vi "ATE_NS_DL_cal.vi"() -> ()   [LabVIEW 2009]
doc: "Use this template to build a producer/consumer design pattern with events to produce queue items. Use this design pattern instead of the User Interface Event Handler pattern for user interfaces when you want to execute code asynchronously in response to an event without slowing the user interface responsiveness."
uses:
  Rvp8PowerData.ctl
panel:
  in  "70 dB Attn":i32=70 min=0 max=70 step=10
  in  "READY":bool
  out "Instructions":string="Noise Source Dummy Load Calibration\n\n1 - Disable or turn off transmitter\n2 - Stow Antenna (point vertically)\n3 - Turn off all florescnt lights\n3 - Start the labview program by clicking the Run arrow\n     (left most button under  drop down menues)\n     start cycle time about 35 seconds\n4 - Wait for the red 'BUSY' light to change to green 'READY'\n     All the control buttons on the control panel are active.\n5 - Select the noise source, its state (ON/OFF) and the wave\n     guide termination.\n6 - Calibrate with the red  'Calibrate' button\n      calibration cycle time is less than 1 minute\n7 - Exit the program with the red 'EXIT' button\n      exit cycle time about 20 seconds\n\nHints:\nWait for the green 'READY' light before clicking buttons\nAll the status leds on the 'Status' tab should be green during a calibration.\nThe antenna noise source does not work with the wave guide\ntermination in the 'Dummy Load' position."
  in  "Configuration 1":bool
  out "Cal Output File":path
  out "Cal file name":string
  in  "Cal data directory":string="/home/operator/ate/data/rvp8_cal"
  in  "Set SigGen":bool
  in  "Initialize":bool
  in  "70 dB":bool
  in  "121 dB":bool
  in  "Switches":bool
  in  "Calibrate":bool
  in  "Stop":bool
  in  "ATE TABS":enum32{"Status", "Controls"}(tab)
  out "ATE Switch Status":T1
  out "RVP8 Power":T2 {"time" format="%<%H:%M:%S\n%Y/%m/%d>T"}
  out "121dB\nAttenuators":bool[](array[boolean])
  out "121 Verified":bool
  out "Inside Noise Box":bool
  in  "WG3 MS":bool
  in  "WG3 T":bool
  out "WG3":bool
  in  "WG2 MS":bool
  in  "WG2 T":bool
  out "WG2":bool
  in  "WG1 MS":bool
  in  "WG1 T":bool
  out "WG1":bool
  in  "WG5 ANT":bool
  in  "WG5 DL":bool
  out "WG5":bool
  in  "WG4 ANT":bool
  in  "WG4 DL":bool
  out "WG4":bool
  out "Outside Noise Box":bool
  out "XmStat":bool=TRUE
  in  "ATE Switches":T3={"Reversing Switch"=enum."Normal Function", "IO Switch #1 Input"=enum."NONE", "IO Switch #1 Output"=enum."NONE", "IO Switch #2 Input"=enum."NONE", "IO Switch #2 Output"=enum."NONE", "Signal Out Input"=enum."NONE", "Signal Out Output"=enum."NONE", "Signal Source Input"=enum."NONE", "Signal Source Output"=enum."NONE", "Power Meter Switch Input"=enum."NONE", "Pouer Meter Switch Output"=enum."NONE", "Amplifier Switch"=enum."Include Amp"}
  in  "DataSource":bool=TRUE
  in  "Measurements":i32=10
  in  "121 dB Atten":i32 min=0 max=121 step=1
  in  "NS_on/off":bool
  in  "Wave Guide Termination":bool
  in  "NoiseSource":u16(ring) items=["Inside Noise Source", "Outside Noise Source", "Agilent Noise Inside", "Agilent Noise Outside"]
  out "P-State":string
  out "C-State":string
  in  "BUSY":bool
  # "ATE Noise Source Calibration"
  # "1 dB"
  # "2 dB"
  # "4 dB"
  # "4 dB"
  # "10 dB"
  # "20 dB"
  # "40 dB"
  # "40 dB"
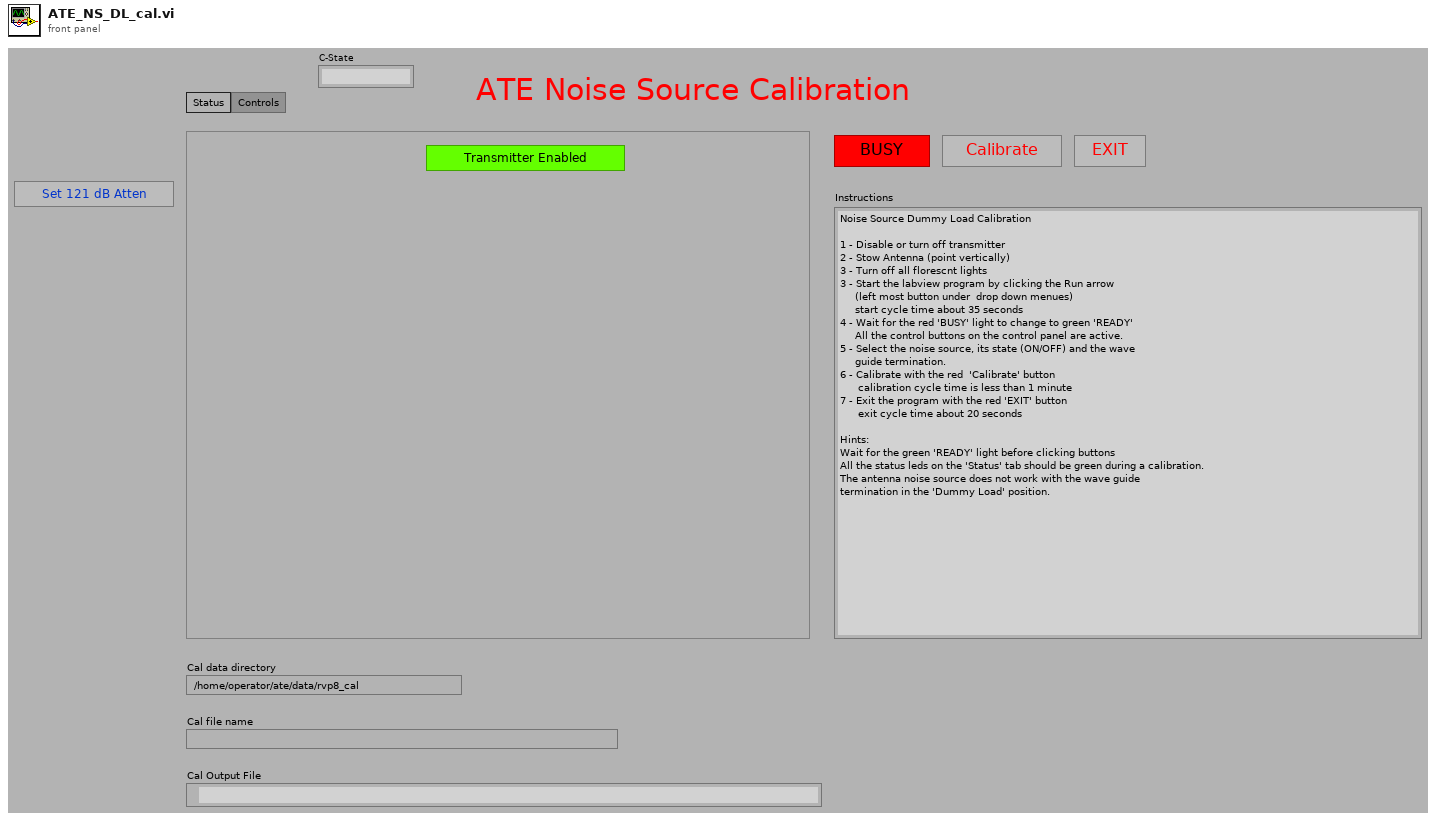
[diagram p1: front panel]
types:
  T1 = cluster{"Reversing Switch ":bool, "IO Switch #1":bool, "IO Switch #2":bool, "Signal Out":bool, "Signal Source":bool, "Power Meter":bool, "Amp By Pass":bool}
  T2 = typedef "Rvp8PowerData.ctl" = cluster{"success":bool, "time":dbl, "el":dbl, "az":dbl, "dbm0":dbl, "dbm1":dbl, "dbmHc":dbl, "dbmHx":dbl, "dbmVc":dbl, "dbmVx":dbl}
  T3 = cluster{"Reversing Switch":enum16{"Normal Function", "Reversing Function"}, "IO Switch #1 Input":enum16{"NONE", "AHR (J2)", "Splitter", "Signal Out Switch (S3)", "Reversing Switch"}, "IO Switch #1 Output":enum16{"NONE", "AHR (J2)", "Delay Device (S4)", "Power Meter Switch (S5)", "Reversing Switch"}, "IO Switch #2 Input":enum16{"NONE", "AVR (J3)", "Splitter", "Signal Out Switch (S3)", " 2W Term (TM1)", "Reversing Switch"}, "IO Switch #2 Output":enum16{"NONE", "AVR (J3)", "Signal Out Switch (S3)", "Power Meter Switch (S5)", "Reversing Switch", "2W Term (TM1)"}, "Signal Out Input":enum16{"NONE", "Amp Bypass Switch (S6)", "IO Switch #1 (S1)", "IO Switch #2 (S2)", "2W Term (TM3)"}, "Signal Out Output":enum16{"NONE", "2 Watt Term (TM3)", "Splitter", "Power Meter Switch (S5)"}, "Signal Source Input":enum16{"NONE", "Delay Device", "Signal Generator (J7)", "Inside Noise Box NF (J5)", "2W Term (TM3)"}, "Signal Source Output":enum16{"NONE", "Amp Bypass Switch", "Test Pulse Generator", "Power Meter Switch (S5)"}, "Power Meter Switch Input":enum16{"NONE", "IO Switch #1 (S1)", "Signal Source Switch (S4)", "Signal Out Switch (S3)", "IO Switch #2 (S2)", "TXH-TXV Switch (J8)"}, "Pouer Meter Switch Output":enum16{"NONE", "Power Meter (J6)"}, "Amplifier Switch":enum16{"Bypass Amp", "Include Amp"}}
  T4 = cluster{"Frequency (GHz)":dbl, "RF Power (dBm)":dbl, "RF ON/OFF":bool}
  T5 = enum16{"open", "replace", "create", "open or create", "replace or create", "replace or create with confirmation"}
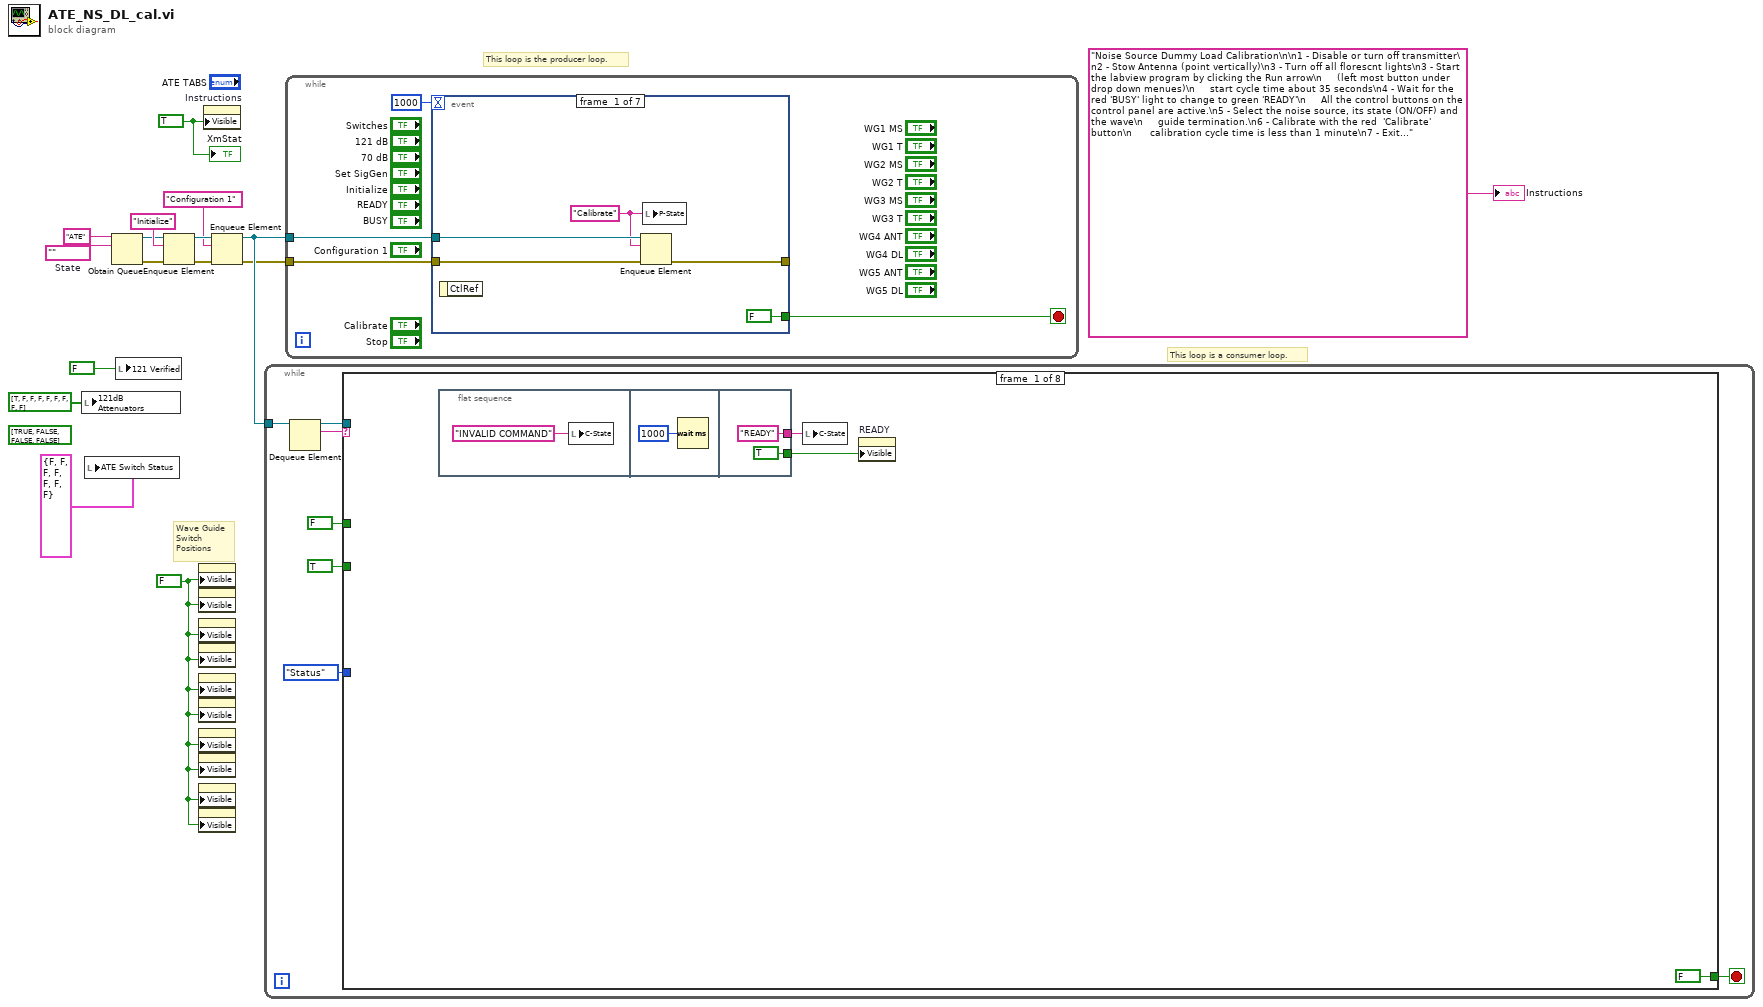
[diagram p0: block diagram]
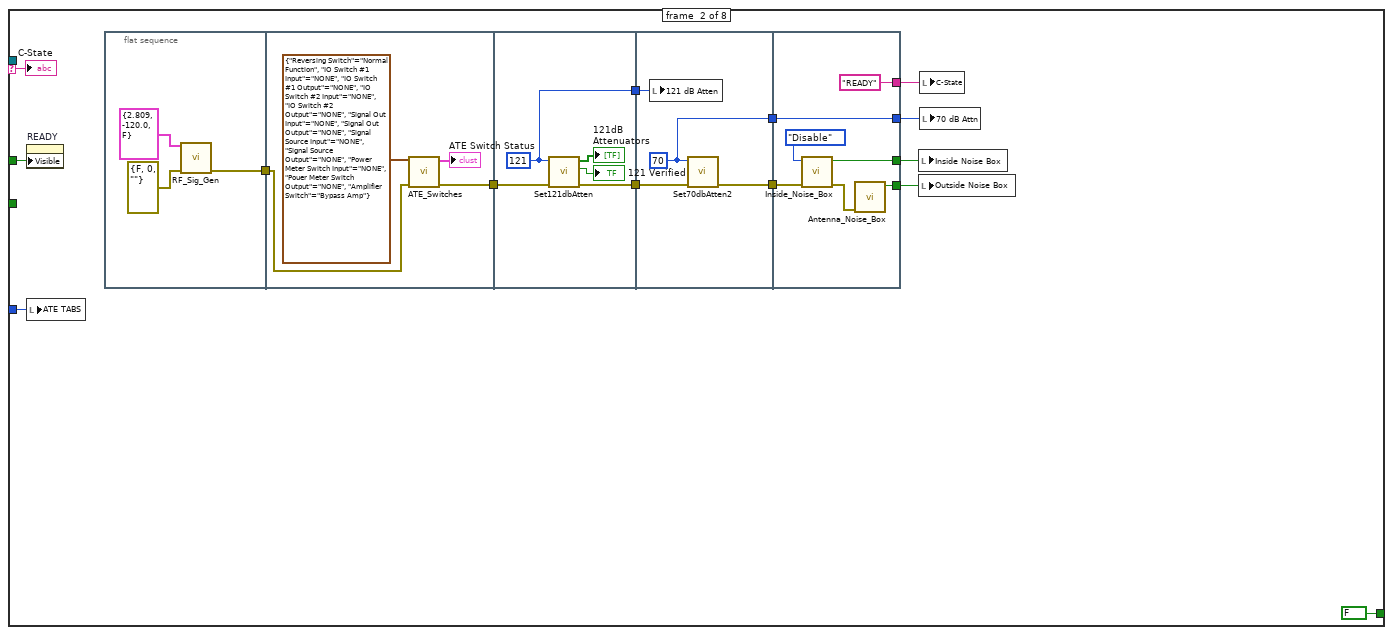
[diagram p2: hidden frame]
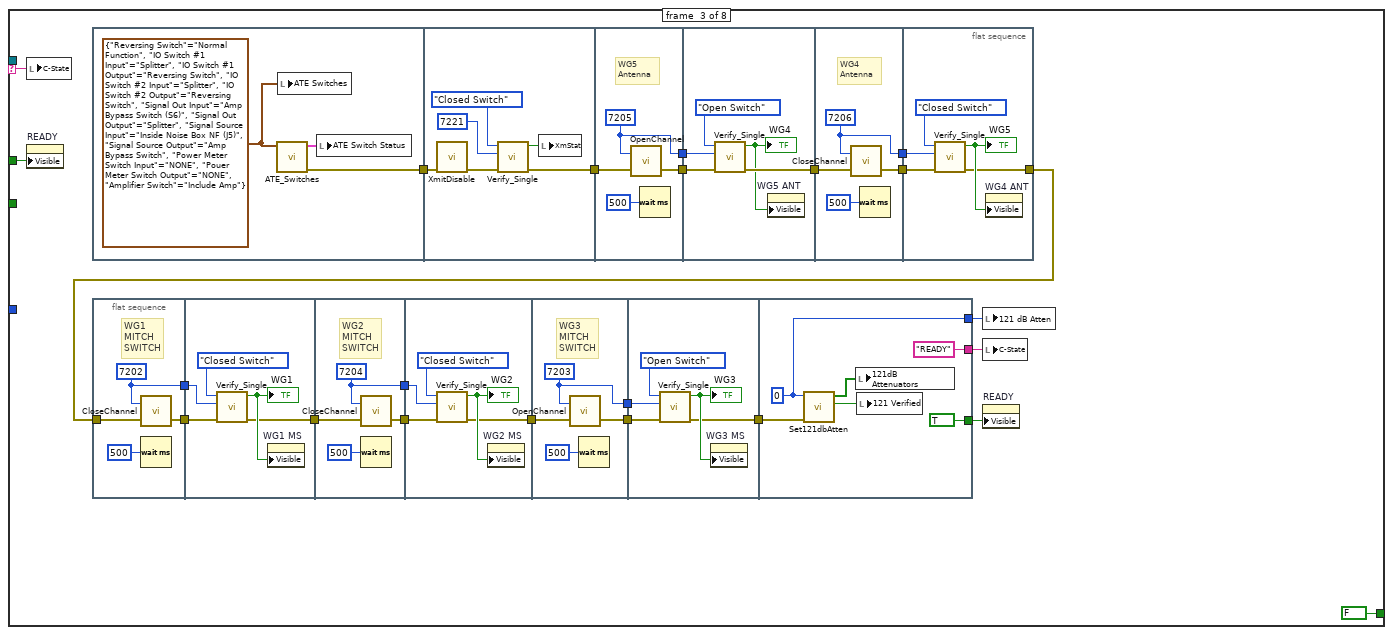
[diagram p3: hidden frame]
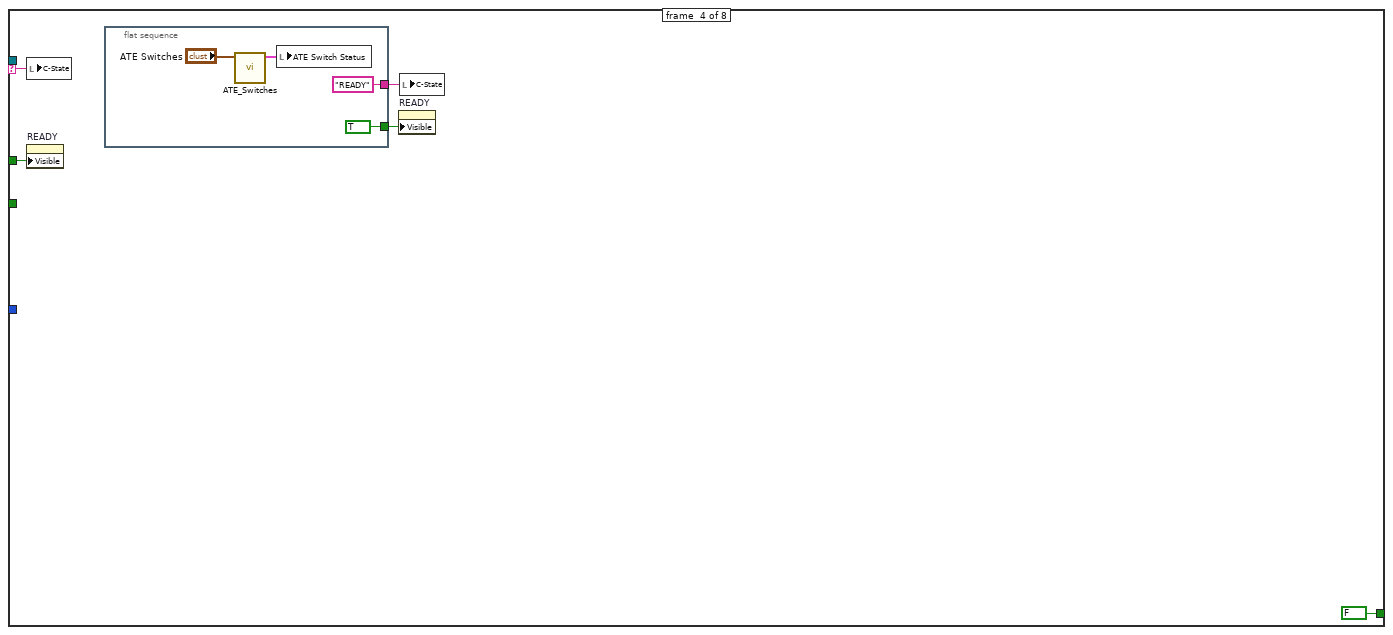
[diagram p4: hidden frame]
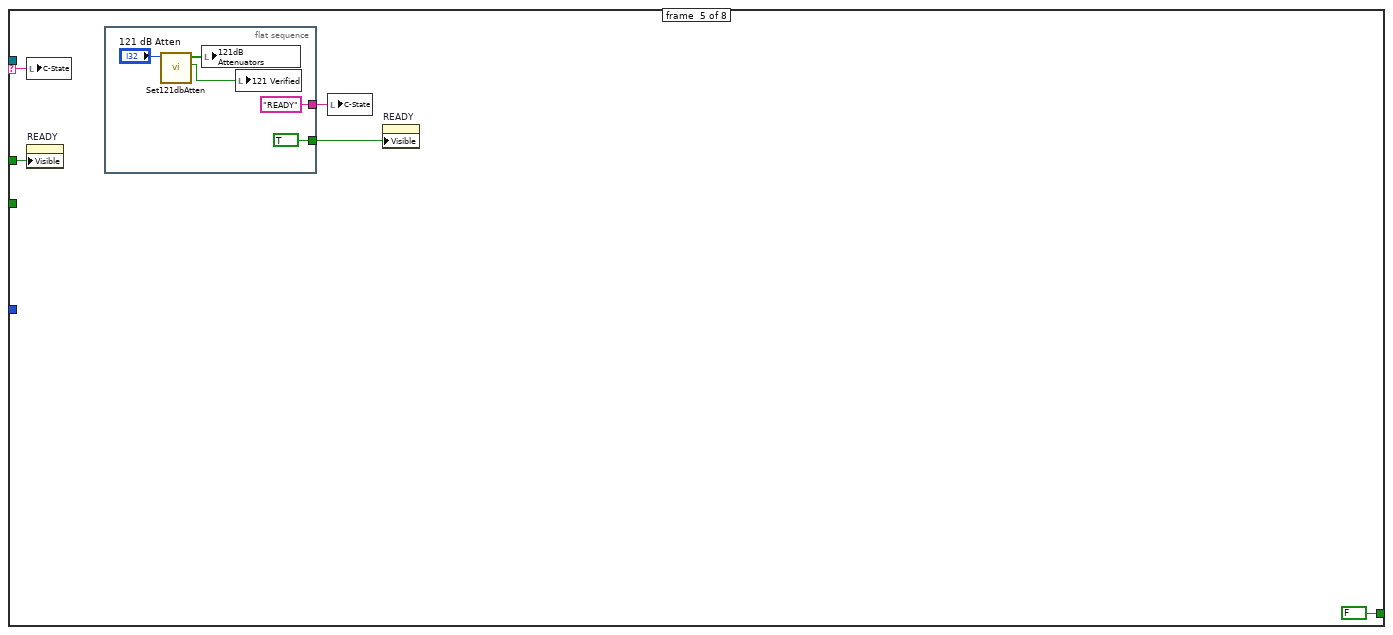
[diagram p5: hidden frame]
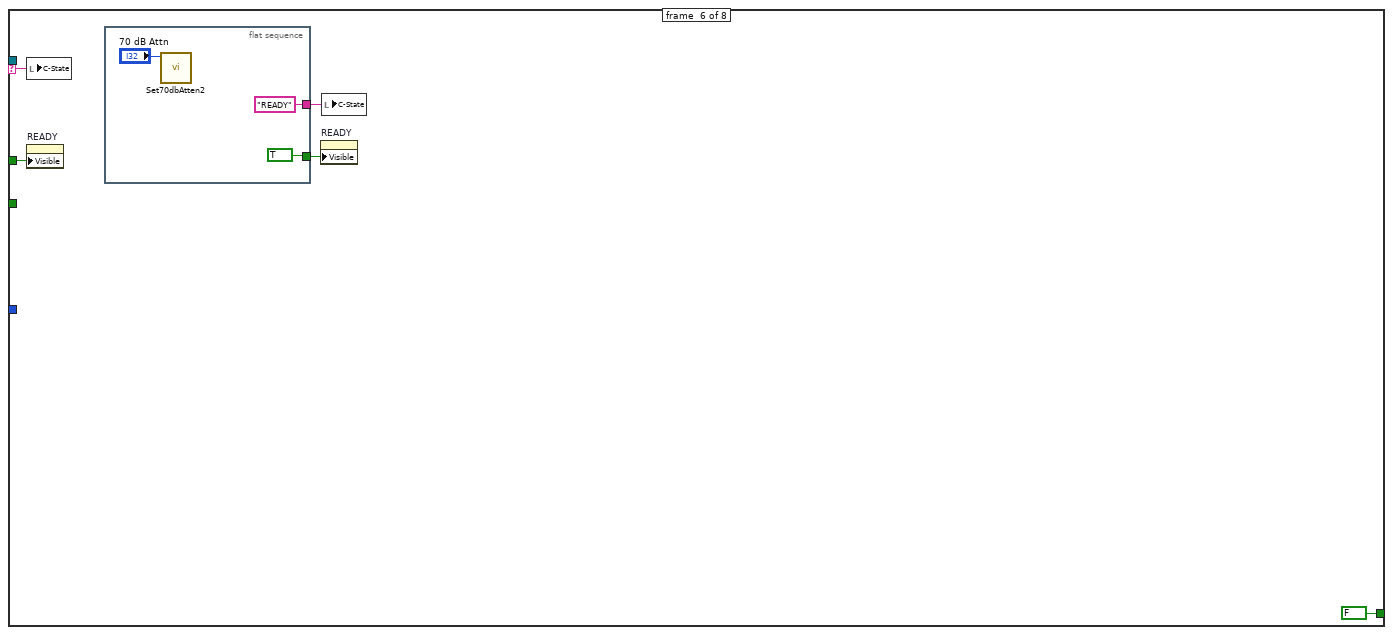
[diagram p6: hidden frame]
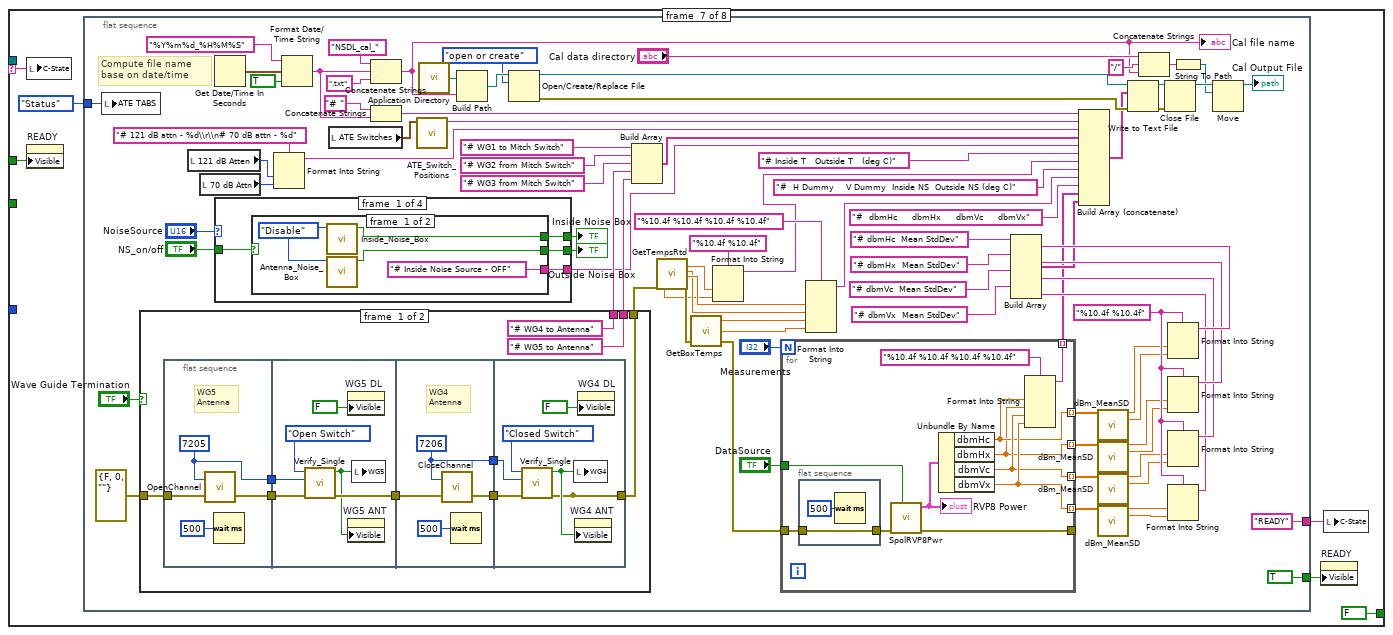
[diagram p7: hidden frame]
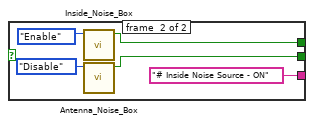
[diagram p8: hidden frame]
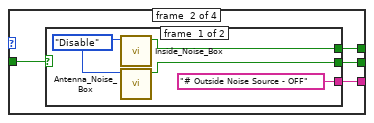
[diagram p9: hidden frame]
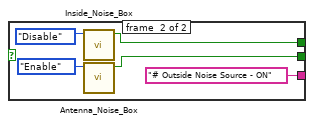
[diagram p10: hidden frame]
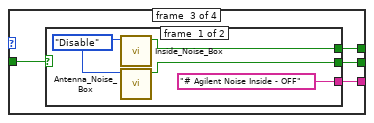
[diagram p11: hidden frame]
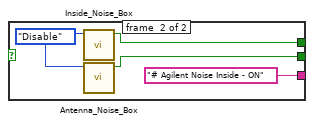
[diagram p12: hidden frame]
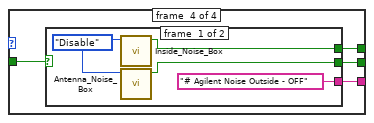
[diagram p13: hidden frame]
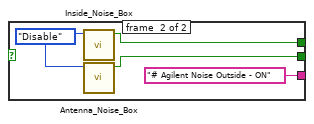
[diagram p14: hidden frame]
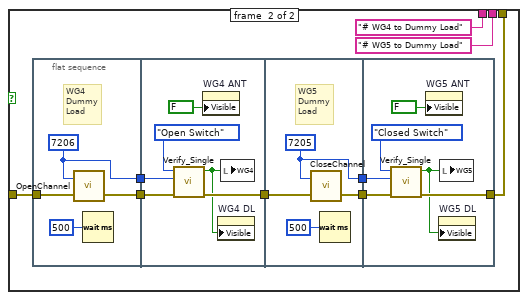
[diagram p15: hidden frame]
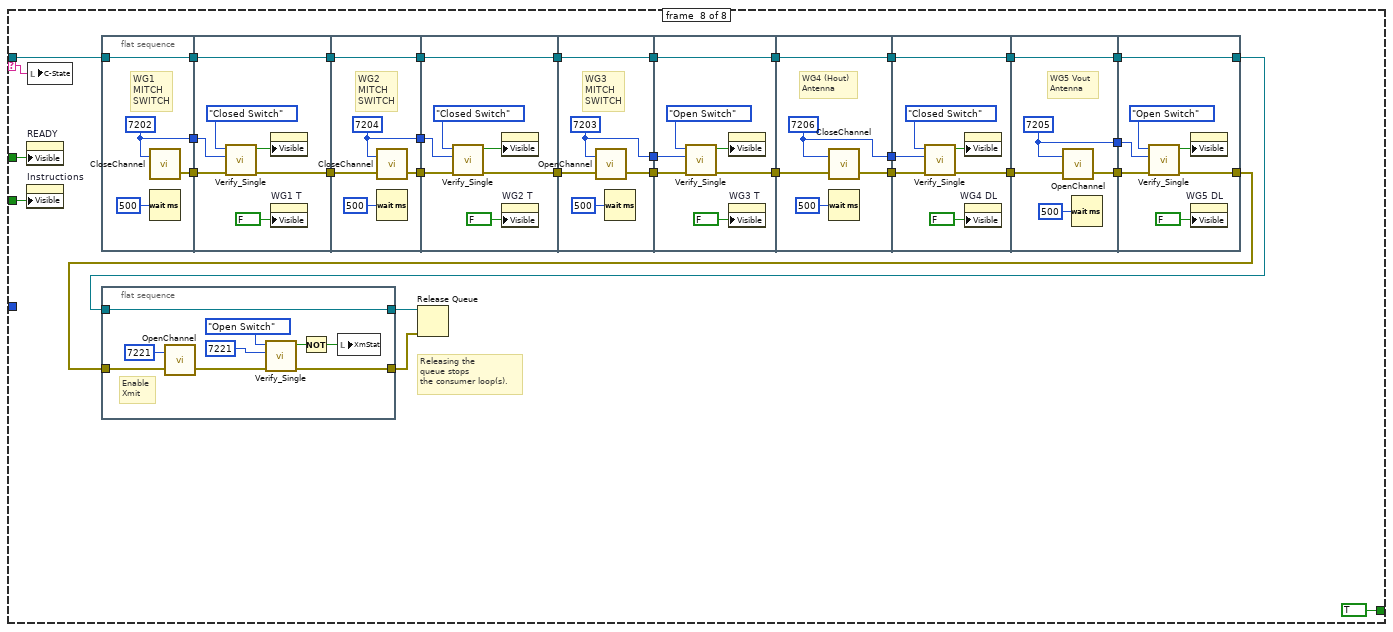
[diagram p16: hidden frame]
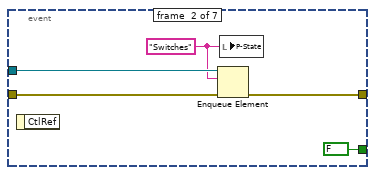
[diagram p17: hidden frame]
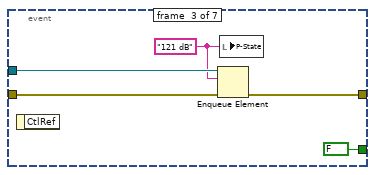
[diagram p18: hidden frame]
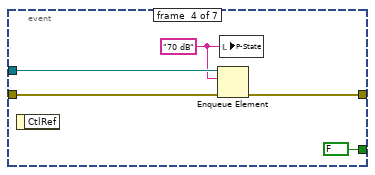
[diagram p19: hidden frame]
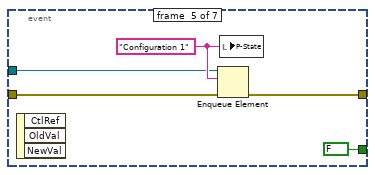
[diagram p20: hidden frame]
diagram:
  w6 = FALSE ("Visible")
  w1 = TRUE ("Visible")
  (unwired) bool[] [TRUE, FALSE, FALSE, FALSE] ("70dB\nAttenuators")
  w16 = ""  # State
  # "Wave Guide\nSwitch\nPositions"
  # "This loop is the producer loop."
  # "This loop is a consumer loop."
  n1 = local write "121dB\nAttenuators"(bool[] [TRUE, FALSE, FALSE, FALSE, FALSE, FALSE, FALSE, FALSE, FALSE] ("121dB\nAttenuators")) -> ()
  n2 = local write "ATE Switch Status"(T1 {"Reversing Switch "=FALSE, "IO Switch #1"=FALSE, "IO Switch #2"=FALSE, "Signal Out"=FALSE, "Signal Source"=FALSE, "Power Meter"=FALSE, "Amp By Pass"=FALSE} ("ATE Switch Status")) -> ()
  n3 = Obtain Queue(name (unnamed)="ATE", element data type=w16) -> (queue out=w13:refnum<queue>, error out=w12:errorcluster)  [unwired: 3 in, 1 out]
  n4 = local write "121 Verified"(FALSE ("70 Verfied")) -> ()
  n5 = Enqueue Element(queue=w13, element="Initialize", error in (no error)=w12) -> (queue out=w7:refnum<queue>, error out=w4:errorcluster)  [unwired: 1 in, 1 out]
  n6 = property on="WG1 MS" class="Bool"("Visible"=w6) -> ()  [unwired: 2 in, 2 out]
  n7 = property on="WG1 T" class="Bool"("Visible"=w6) -> ()  [unwired: 2 in, 2 out]
  n8 = property on="WG2 MS" class="Bool"("Visible"=w6) -> ()  [unwired: 2 in, 2 out]
  n9 = property on="WG2 T" class="Bool"("Visible"=w6) -> ()  [unwired: 2 in, 2 out]
  n10 = property on="WG3 MS" class="Bool"("Visible"=w6) -> ()  [unwired: 2 in, 2 out]
  n11 = property on="WG3 T" class="Bool"("Visible"=w6) -> ()  [unwired: 2 in, 2 out]
  n12 = property on="WG4 ANT" class="Bool"("Visible"=w6) -> ()  [unwired: 2 in, 2 out]
  n13 = property on="WG4 DL" class="Bool"("Visible"=w6) -> ()  [unwired: 2 in, 2 out]
  n14 = property on="WG5 ANT" class="Bool"("Visible"=w6) -> ()  [unwired: 2 in, 2 out]
  n15 = property on="WG5 DL" class="Bool"("Visible"=w6) -> ()  [unwired: 2 in, 2 out]
  n16 = property on="Instructions" class="Str"("Visible"=w1) -> ()  [unwired: 2 in, 2 out]
  n17 = Enqueue Element(queue=w7, element="Configuration 1", error in (no error)=w4) -> (queue out=w5:refnum<queue>, error out=w3:errorcluster)  [unwired: 1 in, 1 out]
  n18 = while {
    tunnel: w5 -> [w23]
    stop <- w20 stop-if-true
    n19 = Dequeue Element(queue=w23) -> (queue out=w21:refnum<queue>, element=w22:string)  [unwired: 2 in, 2 out]
    n20 = case shown="\"Calibrate\"" w22 {
      selector: w22 -> [_ w43 w88 w155 w163 w173 w182 w421]
      tunnel: w21 -> [_ _ _ _ _ _ _ w404]
      tunnel: [FALSE FALSE FALSE FALSE FALSE FALSE FALSE TRUE] -> w20
      tunnel: FALSE ("Visible") -> [_ w37 w87 w152 w161 w171 w180 w420]
      tunnel: TRUE ("Visible") -> [_ _ _ _ _ _ _ w419]
      tunnel: enum32{"Status", "Controls"}."Status" ("ATE TABS") -> [_ w36 _ _ _ _ _ _]
      frame #0 {
        n21 = flat-sequence {
          tunnel: ["READY" ("element")] -> w25
          tunnel: [TRUE ("Visible")] -> w24
          frame #0 {
            n22 = local write "C-State"("INVALID COMMAND" ("C-State")) -> ()
          }
          frame #1 {
            n23 = Wait (ms)(milliseconds to wait=u32 1000) -> ()  [unwired: 1 out]
          }
          frame #2 {
          }
        }
        n24 = local write "C-State"(w25) -> ()
        n25 = property on="READY" class="Bool"("Visible"=w24) -> ()  [unwired: 2 in, 2 out]
      }
      frame #1 {
        n26 = property on="READY" class="Bool"("Visible"=w37) -> ()  [unwired: 2 in, 2 out]
        n27 = local write "ATE TABS"(w36) -> ()
        n28 = flat-sequence {
          tunnel: [w45] -> w38
          tunnel: [w49] -> w41
          tunnel: w38 -> [w50]
          tunnel: w41 -> [w55]
          tunnel: [w54] -> w42
          tunnel: [w53] -> w40
          tunnel: w42 -> [w60]
          tunnel: w40 -> [w59]
          tunnel: [w58] -> w35
          tunnel: [w57] -> w34
          tunnel: [w67] -> w39
          tunnel: w35 -> [w67]
          tunnel: w34 -> [w66]
          tunnel: [w64] -> w33
          tunnel: [w63] -> w32
          tunnel: ["READY" ("element")] -> w31
          frame #0 {
            n29 = call "RF_Sig_Gen.vi"("Signal Generator Control"=T4 {"Frequency (GHz)"=2.809, "RF Power (dBm)"=-120.0, "RF ON/OFF"=FALSE}, "error in"=errorcluster {"status"=FALSE, "code"=0, "source"=""}) -> ("Sig Gen Errors"=w45:errorcluster)  [unwired: 12 in, 1 out]
          }
          frame #1 {
            n30 = call "ATE_Switches.vi"("error in"=w50, "ATE Switches"=T3 {"Reversing Switch"=enum."Normal Function", "IO Switch #1 Input"=enum."NONE", "IO Switch #1 Output"=enum."NONE", "IO Switch #2 Input"=enum."NONE", "IO Switch #2 Output"=enum."NONE", "Signal Out Input"=enum."NONE", "Signal Out Output"=enum."NONE", "Signal Source Input"=enum."NONE", "Signal Source Output"=enum."NONE", "Power Meter Switch Input"=enum."NONE", "Pouer Meter Switch Output"=enum."NONE", "Amplifier Switch"=enum."Bypass Amp"}) -> ("Switch Errors"=w49:errorcluster, "ATE Switch Status"=→"ATE Switch Status":T1)  [unwired: 8 in]
          }
          frame #2 {
            w53 = 121 ("Attenuation (dB)")
            n31 = call "Set121dbAtten.vi"("error in (no error)"=w55, "Attenuation (dB)"=w53) -> ("error out"=w54:errorcluster, "Verfied"=→"121 Verified":bool, "Active Attenuators"=→"121dB\nAttenuators":bool[])  [unwired: 7 in]
          }
          frame #3 {
            w58 = 70 ("Attenuation (dB)")
            n32 = local write "121 dB Atten"(w59) -> ()
            n33 = call "Set70dbAtten2.vi"("error in (no error)"=w60, "Attenuation (dB)"=w58) -> ("error out"=w57:errorcluster)  [unwired: 7 in, 2 out]
          }
          frame #4 {
            n34 = call "Inside_Noise_Box.vi"("error in"=w66, "Noise Switch Function"=enum16{"Disable", "Enable"}."Disable") -> ("error out"=w65:errorcluster, "Verfied"=w64:bool)  [unwired: 8 in]
            n35 = call "Antenna_Noise_Box.vi"("error in"=w65) -> ("Verfied"=w63:bool)  [unwired: 9 in, 1 out]
          }
        }
        n36 = local write "Inside Noise Box"(w33) -> ()
        n37 = local write "Outside Noise Box"(w32) -> ()
        n38 = local write "C-State"(w31) -> ()
        n39 = local write "70 dB Attn"(w39) -> ()
        "C-State" <- w43
      }
      frame #2 {
        n40 = local write "C-State"(w88) -> ()
        n41 = property on="READY" class="Bool"("Visible"=w87) -> ()  [unwired: 2 in, 2 out]
        n42 = flat-sequence {
          tunnel: [w126] -> w89
          tunnel: w89 -> [w132]
          tunnel: [w128] -> w86
          tunnel: w86 -> [w136]
          tunnel: [w135] -> w83
          tunnel: [w134] -> w82
          tunnel: [w138] -> w85
          tunnel: w83 -> [w140]
          tunnel: w82 -> [w139]
          tunnel: [w143] -> w84
          tunnel: w85 -> [w145]
          tunnel: [w142] -> w70
          tunnel: w84 -> [w149]
          tunnel: w70 -> [w148]
          tunnel: [w146] -> w69
          frame #0 {
            w124 = T3 {"Reversing Switch"=enum."Normal Function", "IO Switch #1 Input"=enum."Splitter", "IO Switch #1 Output"=enum."Reversing Switch", "IO Switch #2 Input"=enum."Splitter", "IO Switch #2 Output"=enum."Reversing Switch", "Signal Out Input"=enum."Amp Bypass Switch (S6)", "Signal Out Output"=enum."Splitter", "Signal Source Input"=enum."Inside Noise Box NF (J5)", "Signal Source Output"=enum."Amp Bypass Switch", "Power Meter Switch Input"=enum."NONE", "Pouer Meter Switch Output"=enum."NONE", "Amplifier Switch"=enum."Include Amp"} ("ATE Switches")
            n43 = call "ATE_Switches.vi"("ATE Switches"=w124) -> ("Switch Errors"=w126:errorcluster, "ATE Switch Status"=w125:T1)  [unwired: 9 in]
            n44 = local write "ATE Switches"(w124) -> ()
            n45 = local write "ATE Switch Status"(w125) -> ()
          }
          frame #1 {
            n46 = call "XmitDisable.vi"("error in (no error)"=w132) -> ("error out"=w131:errorcluster)  [unwired: 1 in, 5 out]
            n47 = call "Verify_Single.vi"("error in"=w131, "Switch ID"=7221, "Switch Functin"=enum16{"Open Switch", "Closed Switch"}."Closed Switch") -> ("Error out"=w128:errorcluster, "Verfied"=w127:bool)  [unwired: 7 in]
            n48 = local write "XmStat"(w127) -> ()
          }
          frame #2 {
            w134 = 7205
            # "WG5\nAntenna"
            n49 = call "OpenChannel.vi"("error in (no error)"=w136, "Channel ID"=w134) -> ("error out"=w135:errorcluster)  [unwired: 1 in]
            n50 = Wait (ms)(milliseconds to wait=u32 500) -> ()  [unwired: 1 out]
          }
          frame #3 {
            n51 = call "Verify_Single.vi"("error in"=w140, "Switch ID"=w139, "Switch Functin"=enum16{"Open Switch", "Closed Switch"}."Open Switch") -> ("Error out"=w138:errorcluster, "Verfied"=w137:bool)  [unwired: 7 in]
            "WG4" <- w137
            n52 = property on="WG5 ANT" class="Bool"("Visible"=w137) -> ()  [unwired: 2 in, 2 out]
          }
          frame #4 {
            w142 = 7206
            # "WG4\nAntenna"
            n53 = call "CloseChannel.vi"("error in (no error)"=w145, "Channel ID"=w142) -> ("error out"=w143:errorcluster)  [unwired: 1 in]
            n54 = Wait (ms)(milliseconds to wait=u32 500) -> ()  [unwired: 1 out]
          }
          frame #5 {
            n55 = call "Verify_Single.vi"("error in"=w149, "Switch ID"=w148, "Switch Functin"=enum16{"Open Switch", "Closed Switch"}."Closed Switch") -> ("Error out"=w146:errorcluster, "Verfied"=w147:bool)  [unwired: 7 in]
            "WG5" <- w147
            n56 = property on="WG4 ANT" class="Bool"("Visible"=w147) -> ()  [unwired: 2 in, 2 out]
          }
        }
        n57 = flat-sequence {
          tunnel: [w93] -> w81
          tunnel: [w92] -> w78
          tunnel: w69 -> [w91]
          tunnel: w81 -> [w98]
          tunnel: [w96] -> w80
          tunnel: w78 -> [w95]
          tunnel: w80 -> [w102]
          tunnel: [w101] -> w79
          tunnel: [w100] -> w77
          tunnel: w79 -> [w107]
          tunnel: w77 -> [w106]
          tunnel: [w104] -> w76
          tunnel: w76 -> [w111]
          tunnel: [w110] -> w75
          tunnel: [w109] -> w74
          tunnel: w75 -> [w115]
          tunnel: w74 -> [w116]
          tunnel: [w113] -> w73
          tunnel: w73 -> [w119]
          tunnel: [TRUE ("Visible")] -> w72
          tunnel: ["READY" ("element")] -> w71
          tunnel: [w118] -> w68
          frame #0 {
            w92 = 7202
            # "WG1\nMITCH\nSWITCH"
            n58 = call "CloseChannel.vi"("error in (no error)"=w91, "Channel ID"=w92) -> ("error out"=w93:errorcluster)  [unwired: 1 in]
            n59 = Wait (ms)(milliseconds to wait=u32 500) -> ()  [unwired: 1 out]
          }
          frame #1 {
            n60 = call "Verify_Single.vi"("error in"=w98, "Switch ID"=w95, "Switch Functin"=enum16{"Open Switch", "Closed Switch"}."Closed Switch") -> ("Error out"=w96:errorcluster, "Verfied"=w97:bool)  [unwired: 7 in]
            "WG1" <- w97
            n61 = property on="WG1 MS" class="Bool"("Visible"=w97) -> ()  [unwired: 2 in, 2 out]
          }
          frame #2 {
            w100 = 7204
            # "WG2\nMITCH\nSWITCH"
            n62 = call "CloseChannel.vi"("error in (no error)"=w102, "Channel ID"=w100) -> ("error out"=w101:errorcluster)  [unwired: 1 in]
            n63 = Wait (ms)(milliseconds to wait=u32 500) -> ()  [unwired: 1 out]
          }
          frame #3 {
            n64 = call "Verify_Single.vi"("error in"=w107, "Switch ID"=w106, "Switch Functin"=enum16{"Open Switch", "Closed Switch"}."Closed Switch") -> ("Error out"=w104:errorcluster, "Verfied"=w105:bool)  [unwired: 7 in]
            "WG2" <- w105
            n65 = property on="WG2 MS" class="Bool"("Visible"=w105) -> ()  [unwired: 2 in, 2 out]
          }
          frame #4 {
            w110 = 7203
            # "WG3\nMITCH\nSWITCH"
            n66 = call "OpenChannel.vi"("error in (no error)"=w111, "Channel ID"=w110) -> ("error out"=w109:errorcluster)  [unwired: 1 in]
            n67 = Wait (ms)(milliseconds to wait=u32 500) -> ()  [unwired: 1 out]
          }
          frame #5 {
            n68 = call "Verify_Single.vi"("error in"=w116, "Switch ID"=w115, "Switch Functin"=enum16{"Open Switch", "Closed Switch"}."Open Switch") -> ("Error out"=w113:errorcluster, "Verfied"=w114:bool)  [unwired: 7 in]
            "WG3" <- w114
            n69 = property on="WG3 MS" class="Bool"("Visible"=w114) -> ()  [unwired: 2 in, 2 out]
          }
          frame #6 {
            w118 = 0 ("Attenuation (dB)")
            n70 = call "Set121dbAtten.vi"("error in (no error)"=w119, "Attenuation (dB)"=w118) -> ("Verfied"=w120:bool, "Active Attenuators"=w121:bool[])  [unwired: 7 in, 1 out]
            n71 = local write "121dB\nAttenuators"(w121) -> ()
            n72 = local write "121 Verified"(w120) -> ()
          }
        }
        n73 = local write "121 dB Atten"(w68) -> ()
        n74 = local write "C-State"(w71) -> ()
        n75 = property on="READY" class="Bool"("Visible"=w72) -> ()  [unwired: 2 in, 2 out]
      }
      frame #3 {
        n76 = local write "C-State"(w155) -> ()
        n77 = property on="READY" class="Bool"("Visible"=w152) -> ()  [unwired: 2 in, 2 out]
        n78 = flat-sequence {
          tunnel: ["READY" ("element")] -> w153
          tunnel: [TRUE ("Visible")] -> w151
          frame #0 {
            n79 = call "ATE_Switches.vi"("ATE Switches"="ATE Switches") -> ("ATE Switch Status"=w158:T1)  [unwired: 9 in, 1 out]
            n80 = local write "ATE Switch Status"(w158) -> ()
          }
        }
        n81 = property on="READY" class="Bool"("Visible"=w151) -> ()  [unwired: 2 in, 2 out]
        n82 = local write "C-State"(w153) -> ()
      }
      frame #4 {
        n83 = local write "C-State"(w163) -> ()
        n84 = property on="READY" class="Bool"("Visible"=w161) -> ()  [unwired: 2 in, 2 out]
        n85 = flat-sequence {
          tunnel: ["READY" ("element")] -> w162
          tunnel: [TRUE ("Visible")] -> w160
          frame #0 {
            n86 = call "Set121dbAtten.vi"("Attenuation (dB)"="121 dB Atten") -> ("Verfied"=w166:bool, "Active Attenuators"=w168:bool[])  [unwired: 8 in, 1 out]
            n87 = local write "121dB\nAttenuators"(w168) -> ()
            n88 = local write "121 Verified"(w166) -> ()
          }
        }
        n89 = local write "C-State"(w162) -> ()
        n90 = property on="READY" class="Bool"("Visible"=w160) -> ()  [unwired: 2 in, 2 out]
      }
      frame #5 {
        n91 = local write "C-State"(w173) -> ()
        n92 = property on="READY" class="Bool"("Visible"=w171) -> ()  [unwired: 2 in, 2 out]
        n93 = flat-sequence {
          tunnel: ["READY" ("element")] -> w172
          tunnel: [TRUE ("Visible")] -> w170
          frame #0 {
            n94 = call "Set70dbAtten2.vi"("Attenuation (dB)"="70 dB Attn") -> ()  [unwired: 8 in, 3 out]
          }
        }
        n95 = property on="READY" class="Bool"("Visible"=w170) -> ()  [unwired: 2 in, 2 out]
        n96 = local write "C-State"(w172) -> ()
      }
      frame #6 {
        n97 = local write "C-State"(w182) -> ()
        n98 = property on="READY" class="Bool"("Visible"=w180) -> ()  [unwired: 2 in, 2 out]
        n99 = flat-sequence {
          tunnel: ["READY" ("element")] -> w181
          tunnel: [TRUE ("Visible")] -> w179
          tunnel: enum32{"Status", "Controls"}."Status" ("ATE TABS") -> [w237]
          frame #0 {
            w209 = "%10.4f %10.4f"
            # "Compute file name base on date/time"
            n100 = local write "ATE TABS"(w237) -> ()
            n101 = case shown="True" "Wave Guide Termination" {
              tunnel: errorcluster {"status"=FALSE, "code"=0, "source"=""} ("error out") -> [w323 w352]
              tunnel: [w322 w351] -> w224
              tunnel: ["# WG4 to Antenna" "# WG4 to Dummy Load"] -> w231
              tunnel: ["# WG5 to Antenna" "# WG5 to Dummy Load"] -> w230
              frame #0 {
                n102 = flat-sequence {
                  tunnel: [w331] -> w328
                  tunnel: [w330] -> w327
                  tunnel: w323 -> [w329]
                  tunnel: w328 -> [w337]
                  tunnel: [w336] -> w326
                  tunnel: w327 -> [w335]
                  tunnel: w326 -> [w341]
                  tunnel: [w340] -> w325
                  tunnel: [w339] -> w324
                  tunnel: w325 -> [w347]
                  tunnel: [w343] -> _
                  tunnel: w324 -> [w346]
                  tunnel: [w343] -> w322
                  frame #0 {
                    w330 = 7205
                    # "WG5\nAntenna"
                    n103 = call "OpenChannel.vi"("error in (no error)"=w329, "Channel ID"=w330) -> ("error out"=w331:errorcluster)  [unwired: 1 in]
                    n104 = Wait (ms)(milliseconds to wait=u32 500) -> ()  [unwired: 1 out]
                  }
                  frame #1 {
                    n105 = call "Verify_Single.vi"("error in"=w337, "Switch ID"=w335, "Switch Functin"=enum16{"Open Switch", "Closed Switch"}."Open Switch") -> ("Error out"=w336:errorcluster, "Verfied"=w334:bool)  [unwired: 7 in]
                    n106 = property on="WG5 DL" class="Bool"("Visible"=FALSE) -> ()  [unwired: 2 in, 2 out]
                    n107 = property on="WG5 ANT" class="Bool"("Visible"=w334) -> ()  [unwired: 2 in, 2 out]
                    n108 = local write "WG5"(w334) -> ()
                  }
                  frame #2 {
                    w339 = 7206
                    # "WG4\nAntenna"
                    n109 = call "CloseChannel.vi"("error in (no error)"=w341, "Channel ID"=w339) -> ("error out"=w340:errorcluster)  [unwired: 1 in]
                    n110 = Wait (ms)(milliseconds to wait=u32 500) -> ()  [unwired: 1 out]
                  }
                  frame #3 {
                    n111 = call "Verify_Single.vi"("error in"=w347, "Switch ID"=w346, "Switch Functin"=enum16{"Open Switch", "Closed Switch"}."Closed Switch") -> ("Error out"=w343:errorcluster, "Verfied"=w345:bool)  [unwired: 7 in]
                    n112 = local write "WG4"(w345) -> ()
                    n113 = property on="WG4 ANT" class="Bool"("Visible"=w345) -> ()  [unwired: 2 in, 2 out]
                    n114 = property on="WG4 DL" class="Bool"("Visible"=FALSE) -> ()  [unwired: 2 in, 2 out]
                  }
                }
              }
              frame #1 {
                n115 = flat-sequence {
                  tunnel: [w360] -> w357
                  tunnel: [w359] -> w356
                  tunnel: w352 -> [w358]
                  tunnel: w357 -> [w366]
                  tunnel: [w365] -> w355
                  tunnel: w356 -> [w364]
                  tunnel: w355 -> [w370]
                  tunnel: [w369] -> w354
                  tunnel: [w368] -> w353
                  tunnel: w354 -> [w376]
                  tunnel: [w375] -> w351
                  tunnel: w353 -> [w374]
                  frame #0 {
                    w359 = 7206
                    # "WG4\nDummy\nLoad"
                    n116 = call "OpenChannel.vi"("error in (no error)"=w358, "Channel ID"=w359) -> ("error out"=w360:errorcluster)  [unwired: 1 in]
                    n117 = Wait (ms)(milliseconds to wait=u32 500) -> ()  [unwired: 1 out]
                  }
                  frame #1 {
                    n118 = call "Verify_Single.vi"("error in"=w366, "Switch ID"=w364, "Switch Functin"=enum16{"Open Switch", "Closed Switch"}."Open Switch") -> ("Error out"=w365:errorcluster, "Verfied"=w363:bool)  [unwired: 7 in]
                    n119 = property on="WG4 ANT" class="Bool"("Visible"=FALSE) -> ()  [unwired: 2 in, 2 out]
                    n120 = property on="WG4 DL" class="Bool"("Visible"=w363) -> ()  [unwired: 2 in, 2 out]
                    n121 = local write "WG4"(w363) -> ()
                  }
                  frame #2 {
                    w368 = 7205
                    # "WG5\nDummy\nLoad"
                    n122 = call "CloseChannel.vi"("error in (no error)"=w370, "Channel ID"=w368) -> ("error out"=w369:errorcluster)  [unwired: 1 in]
                    n123 = Wait (ms)(milliseconds to wait=u32 500) -> ()  [unwired: 1 out]
                  }
                  frame #3 {
                    n124 = call "Verify_Single.vi"("error in"=w376, "Switch ID"=w374, "Switch Functin"=enum16{"Open Switch", "Closed Switch"}."Closed Switch") -> ("Error out"=w375:errorcluster, "Verfied"=w373:bool)  [unwired: 7 in]
                    n125 = property on="WG5 ANT" class="Bool"("Visible"=FALSE) -> ()  [unwired: 2 in, 2 out]
                    n126 = property on="WG5 DL" class="Bool"("Visible"=w373) -> ()  [unwired: 2 in, 2 out]
                    n127 = local write "WG5"(w373) -> ()
                  }
                }
              }
            }
            n128 = local read "121 dB Atten"() -> (w251:i32)
            n129 = local read "70 dB Attn"() -> (w250:i32)
            n130 = Get Date/Time In Seconds() -> (seconds since 1Jan1904=w264:timestamp)
            n131 = case shown="1" "NoiseSource" {
              tunnel: "NS_on/off" -> [w272 w284 w299 w311]
              tunnel: [w273 w286 w298 w310] -> w210
              tunnel: [w271 w285 w297 w309] -> w227
              tunnel: [w270 w283 w296 w308] -> w207
              frame #0 {
                n132 = case shown="True" w272 {
                  tunnel: ["# Inside Noise Source - OFF" "# Inside Noise Source - ON"] -> w273
                  tunnel: [w275 w279] -> w271
                  tunnel: [w274 w278] -> w270
                  frame #0 {
                    w276 = enum16{"Disable", "Enable"}."Disable" ("Noise Switch Function")
                    n133 = call "Inside_Noise_Box.vi"("Noise Switch Function"=w276) -> ("Verfied"=w275:bool)  [unwired: 9 in, 1 out]
                    n134 = call "Antenna_Noise_Box.vi"("Noise Switch Function"=w276) -> ("Verfied"=w274:bool)  [unwired: 9 in, 1 out]
                  }
                  frame #1 {
                    n135 = call "Inside_Noise_Box.vi"("Noise Switch Function"=enum16{"Disable", "Enable"}."Enable") -> ("Verfied"=w279:bool)  [unwired: 9 in, 1 out]
                    n136 = call "Antenna_Noise_Box.vi"("Noise Switch Function"=enum16{"Disable", "Enable"}."Disable") -> ("Verfied"=w278:bool)  [unwired: 9 in, 1 out]
                  }
                }
              }
              frame #1 {
                n137 = case shown="False" w284 {
                  tunnel: ["# Outside Noise Source - OFF" "# Outside Noise Source - ON"] -> w286
                  tunnel: [w288 w292] -> w285
                  tunnel: [w287 w291] -> w283
                  frame #0 {
                    w289 = enum16{"Disable", "Enable"}."Disable" ("Noise Switch Function")
                    n138 = call "Inside_Noise_Box.vi"("Noise Switch Function"=w289) -> ("Verfied"=w288:bool)  [unwired: 9 in, 1 out]
                    n139 = call "Antenna_Noise_Box.vi"("Noise Switch Function"=w289) -> ("Verfied"=w287:bool)  [unwired: 9 in, 1 out]
                  }
                  frame #1 {
                    n140 = call "Inside_Noise_Box.vi"("Noise Switch Function"=enum16{"Disable", "Enable"}."Disable") -> ("Verfied"=w292:bool)  [unwired: 9 in, 1 out]
                    n141 = call "Antenna_Noise_Box.vi"("Noise Switch Function"=enum16{"Disable", "Enable"}."Enable") -> ("Verfied"=w291:bool)  [unwired: 9 in, 1 out]
                  }
                }
              }
              frame #2 {
                n142 = case shown="True" w299 {
                  tunnel: ["# Agilent Noise Inside - OFF" "# Agilent Noise Inside - ON"] -> w298
                  tunnel: [w301 w305] -> w297
                  tunnel: [w300 w304] -> w296
                  frame #0 {
                    w302 = enum16{"Disable", "Enable"}."Disable" ("Noise Switch Function")
                    n143 = call "Inside_Noise_Box.vi"("Noise Switch Function"=w302) -> ("Verfied"=w301:bool)  [unwired: 9 in, 1 out]
                    n144 = call "Antenna_Noise_Box.vi"("Noise Switch Function"=w302) -> ("Verfied"=w300:bool)  [unwired: 9 in, 1 out]
                  }
                  frame #1 {
                    w306 = enum16{"Disable", "Enable"}."Disable" ("Noise Switch Function")
                    n145 = call "Inside_Noise_Box.vi"("Noise Switch Function"=w306) -> ("Verfied"=w305:bool)  [unwired: 9 in, 1 out]
                    n146 = call "Antenna_Noise_Box.vi"("Noise Switch Function"=w306) -> ("Verfied"=w304:bool)  [unwired: 9 in, 1 out]
                  }
                }
              }
              frame #3 {
                n147 = case shown="False" w311 {
                  tunnel: ["# Agilent Noise Outside - OFF" "# Agilent Noise Outside - ON"] -> w310
                  tunnel: [w313 w317] -> w309
                  tunnel: [w312 w316] -> w308
                  frame #0 {
                    w314 = enum16{"Disable", "Enable"}."Disable" ("Noise Switch Function")
                    n148 = call "Inside_Noise_Box.vi"("Noise Switch Function"=w314) -> ("Verfied"=w313:bool)  [unwired: 9 in, 1 out]
                    n149 = call "Antenna_Noise_Box.vi"("Noise Switch Function"=w314) -> ("Verfied"=w312:bool)  [unwired: 9 in, 1 out]
                  }
                  frame #1 {
                    w318 = enum16{"Disable", "Enable"}."Disable" ("Noise Switch Function")
                    n150 = call "Inside_Noise_Box.vi"("Noise Switch Function"=w318) -> ("Verfied"=w317:bool)  [unwired: 9 in, 1 out]
                    n151 = call "Antenna_Noise_Box.vi"("Noise Switch Function"=w318) -> ("Verfied"=w316:bool)  [unwired: 9 in, 1 out]
                  }
                }
              }
            }
            "Inside Noise Box" <- w227
            "Outside Noise Box" <- w207
            n152 = Format Into String(format string="# 121 dB attn - %d\\r\\n# 70 dB attn - %d", w251, w250) -> (resulting string=w245:string)  [unwired: 2 in, 1 out]
            n153 = Format Date/Time String(time format string (%c)="%Y%m%d_%H%M%S", seconds (now)=w264, UTC format=TRUE) -> (date/time string=w240:string)
            n154 = local read "ATE Switches"() -> (w244:T3)
            n155 = Concatenate Strings("NSDL_cal_", w240, ".txt") -> (w239:string)
            "Cal file name" <- w239
            n156 = Concatenate Strings("# " ("string"), w240) -> (w247:string)
            n157 = call "ATE_Switch_Positions.vi"("ATE Switches"=w244) -> ("ATE Switch/Position"=w246:string)  [unwired: 10 in]
            n158 = call <vilib>:"Application Directory.vi"() -> ("Application Directory"=w241:path)
            n159 = Build Path(base path=w241, name or relative path=w239) -> (appended path=w263:path)
            n160 = Open/Create/Replace File(file path (use dialog)=w263, operation (0:open)=T5."open or create") -> (refnum out=w262:refnum<file>, error out=w261:errorcluster)  [unwired: 4 in, 1 out]
            n161 = Build Array("# WG1 to Mitch Switch", "# WG2 from Mitch Switch", "# WG3 from Mitch Switch", w231, w230) -> (w229:string[])
            n162 = call "GetTempsRtd.vi"("error in (no error)"=w224) -> ("Temp Outside"=w198:dbl, "Temp Inside"=w199:dbl, "Temp V Dummy"=w225:dbl, "Temp H Dummy"=w226:dbl, "error out"=w223:errorcluster)  [unwired: 2 in, 12 out]
            n163 = call "GetBoxTemps.vi"("error in (no error)"=w223) -> ("error out"=w222:errorcluster, "Outside Box"=w206:dbl, "InsideBox"=w221:dbl)  [unwired: 1 in, 1 out]
            n164 = Format Into String(format string="%10.4f %10.4f", w199, w198) -> (resulting string=w196:string)  [unwired: 2 in, 1 out]
            n165 = for {
              N: "Measurements" -> [_]
              tunnel: w222 -> [w382]
              tunnel: [w388] -> w204 mode=indexing
              tunnel: [w383] -> _
              tunnel: "DataSource" -> [w385]
              tunnel: [w381] -> w192 mode=indexing
              tunnel: [w380] -> w193 mode=indexing
              tunnel: [w378] -> w194 mode=indexing
              tunnel: [w379] -> w195 mode=indexing
              n166 = flat-sequence {
                tunnel: w382 -> [w390]
                tunnel: [w390] -> w387
                frame #0 {
                  n167 = Wait (ms)(milliseconds to wait=u32 500) -> ()  [unwired: 1 out]
                }
              }
              n168 = call "SpolRVP8Pwr.vi"("DataSource"=w385, "error in (no error)"=w387) -> ("Comm error"=w383:errorcluster, "RVP8_power"=w384:T2)  [unwired: 6 in, 2 out]
              "RVP8 Power" <- w384
              n169 = Unbundle By Name(w384) -> ("dbmHc"=w379:dbl, "dbmHx"=w378:dbl, "dbmVc"=w380:dbl, "dbmVx"=w381:dbl)
              n170 = Format Into String(format string="%10.4f %10.4f %10.4f %10.4f", w379, w378, w380, w381) -> (resulting string=w388:string)  [unwired: 2 in, 1 out]
            }
            n171 = Format Into String(format string="%10.4f %10.4f %10.4f %10.4f", w226, w225, w221, w206) -> (resulting string=w201:string)  [unwired: 2 in, 1 out]
            n172 = call "dBm_MeanSD.vi"("dBm array"=w195) -> ("dBm mean"=w191:dbl, "Std Dev"=w190:dbl)  [unwired: 13 in]
            n173 = call "dBm_MeanSD.vi"("dBm array"=w194) -> ("dBm mean"=w189:dbl, "Std Dev"=w188:dbl)  [unwired: 13 in]
            n174 = call "dBm_MeanSD.vi"("dBm array"=w193) -> ("dBm mean"=w187:dbl, "Std Dev"=w186:dbl)  [unwired: 13 in]
            n175 = call "dBm_MeanSD.vi"("dBm array"=w192) -> ("dBm mean"=w185:dbl, "Std Dev"=w184:dbl)  [unwired: 13 in]
            n176 = Concatenate Strings("Cal data directory", "/" ("string"), w239) -> (w257:string)
            n177 = Format Into String(format string=w209, w191, w190) -> (resulting string=w215:string)  [unwired: 2 in, 1 out]
            n178 = Format Into String(format string=w209, w189, w188) -> (resulting string=w214:string)  [unwired: 2 in, 1 out]
            n179 = Format Into String(format string=w209, w187, w186) -> (resulting string=w213:string)  [unwired: 2 in, 1 out]
            n180 = Format Into String(format string=w209, w185, w184) -> (resulting string=w212:string)  [unwired: 2 in, 1 out]
            n181 = Build Array("# dbmHc  Mean StdDev", w215, "# dbmHx  Mean StdDev", w214, "# dbmVc  Mean StdDev", w213, "# dbmVx  Mean StdDev", w212) -> (w205:string[])
            n182 = Build Array (concatenate)(w247, w246, w245, w229, w210, "# Inside T   Outside T   (deg C)", w196, "#  H Dummy    V Dummy  Inside NS  Outside NS (deg C)", w201, "#  dbmHc     dbmHx     dbmVc     dbmVx", w204, w205) -> (w253:string[])
            n183 = Write to Text File(file (use dialog)=w262, text=w253, error in=w261) -> (refnum out=w260:refnum<file>, error out=w259:errorcluster)  [unwired: 1 in, 1 out]
            n184 = Close File(refnum=w260, error in=w259) -> (path=w256:path)  [unwired: 1 out]
            n185 = String To Path(string=w257) -> (path=w255:path)
            n186 = Move(source path=w256, 10:w255) -> (3:→"Cal Output File":path)  [unwired: 3 in, 2 out]
          }
        }
        n187 = property on="READY" class="Bool"("Visible"=w179) -> ()  [unwired: 2 in, 2 out]
        n188 = local write "C-State"(w181) -> ()
      }
      frame #7 {
        # "Releasing the\nqueue stops\nthe consumer loop(s)."
        n189 = property on="READY" class="Bool"("Visible"=w420) -> ()  [unwired: 2 in, 2 out]
        n190 = property on="Instructions" class="Str"("Visible"=w419) -> ()  [unwired: 2 in, 2 out]
        n191 = local write "C-State"(w421) -> ()
        n192 = flat-sequence {
          tunnel: [w434] -> w418
          tunnel: [w433] -> w417
          tunnel: w404 -> [w432]
          tunnel: [w432] -> w395
          tunnel: w418 -> [w441]
          tunnel: [w440] -> w416
          tunnel: w417 -> [w439]
          tunnel: [w438] -> w396
          tunnel: w395 -> [w438]
          tunnel: w416 -> [w446]
          tunnel: [w445] -> w415
          tunnel: [w444] -> w414
          tunnel: [w443] -> w397
          tunnel: w396 -> [w443]
          tunnel: w415 -> [w453]
          tunnel: w414 -> [w452]
          tunnel: [w451] -> w413
          tunnel: [w450] -> w398
          tunnel: w397 -> [w450]
          tunnel: w413 -> [w458]
          tunnel: [w457] -> w412
          tunnel: [w456] -> w411
          tunnel: [w455] -> w399
          tunnel: w398 -> [w455]
          tunnel: w412 -> [w464]
          tunnel: w411 -> [w465]
          tunnel: [w463] -> w410
          tunnel: [w462] -> w400
          tunnel: w399 -> [w462]
          tunnel: w410 -> [w470]
          tunnel: [w469] -> w409
          tunnel: [w468] -> w407
          tunnel: [w467] -> w401
          tunnel: w400 -> [w467]
          tunnel: w409 -> [w475]
          tunnel: [w476] -> w408
          tunnel: w407 -> [w477]
          tunnel: [w474] -> w402
          tunnel: w401 -> [w474]
          tunnel: w408 -> [w482]
          tunnel: [w481] -> w406
          tunnel: [w480] -> w405
          tunnel: [w479] -> w403
          tunnel: w402 -> [w479]
          tunnel: w406 -> [w489]
          tunnel: w405 -> [w488]
          tunnel: [w487] -> w394
          tunnel: w403 -> [w487]
          tunnel: [w484] -> w392
          frame #0 {
            w433 = 7202
            # "WG1\nMITCH\nSWITCH"
            n193 = call "CloseChannel.vi"("Channel ID"=w433) -> ("error out"=w434:errorcluster)  [unwired: 2 in]
            n194 = Wait (ms)(milliseconds to wait=u32 500) -> ()  [unwired: 1 out]
          }
          frame #1 {
            n195 = call "Verify_Single.vi"("error in"=w441, "Switch ID"=w439, "Switch Functin"=enum16{"Open Switch", "Closed Switch"}."Closed Switch") -> ("Error out"=w440:errorcluster, "Verfied"=w437:bool)  [unwired: 7 in]
            n196 = property on="WG1 MS" class="Bool"("Visible"=w437) -> ()  [unwired: 2 in, 2 out]
            n197 = property on="WG1 T" class="Bool"("Visible"=FALSE) -> ()  [unwired: 2 in, 2 out]
          }
          frame #2 {
            w444 = 7204
            # "WG2\nMITCH\nSWITCH"
            n198 = call "CloseChannel.vi"("error in (no error)"=w446, "Channel ID"=w444) -> ("error out"=w445:errorcluster)  [unwired: 1 in]
            n199 = Wait (ms)(milliseconds to wait=u32 500) -> ()  [unwired: 1 out]
          }
          frame #3 {
            n200 = call "Verify_Single.vi"("error in"=w453, "Switch ID"=w452, "Switch Functin"=enum16{"Open Switch", "Closed Switch"}."Closed Switch") -> ("Error out"=w451:errorcluster, "Verfied"=w449:bool)  [unwired: 7 in]
            n201 = property on="WG2 MS" class="Bool"("Visible"=w449) -> ()  [unwired: 2 in, 2 out]
            n202 = property on="WG2 T" class="Bool"("Visible"=FALSE) -> ()  [unwired: 2 in, 2 out]
          }
          frame #4 {
            w457 = 7203
            # "WG3\nMITCH\nSWITCH"
            n203 = call "OpenChannel.vi"("error in (no error)"=w458, "Channel ID"=w457) -> ("error out"=w456:errorcluster)  [unwired: 1 in]
            n204 = Wait (ms)(milliseconds to wait=u32 500) -> ()  [unwired: 1 out]
          }
          frame #5 {
            n205 = call "Verify_Single.vi"("error in"=w465, "Switch ID"=w464, "Switch Functin"=enum16{"Open Switch", "Closed Switch"}."Open Switch") -> ("Error out"=w463:errorcluster, "Verfied"=w461:bool)  [unwired: 7 in]
            n206 = property on="WG3 MS" class="Bool"("Visible"=w461) -> ()  [unwired: 2 in, 2 out]
            n207 = property on="WG3 T" class="Bool"("Visible"=FALSE) -> ()  [unwired: 2 in, 2 out]
          }
          frame #6 {
            w468 = 7206
            # "WG4 (Hout)\nAntenna"
            n208 = call "CloseChannel.vi"("error in (no error)"=w470, "Channel ID"=w468) -> ("error out"=w469:errorcluster)  [unwired: 1 in]
            n209 = Wait (ms)(milliseconds to wait=u32 500) -> ()  [unwired: 1 out]
          }
          frame #7 {
            n210 = call "Verify_Single.vi"("error in"=w475, "Switch ID"=w477, "Switch Functin"=enum16{"Open Switch", "Closed Switch"}."Closed Switch") -> ("Error out"=w476:errorcluster, "Verfied"=w473:bool)  [unwired: 7 in]
            n211 = property on="WG4 ANT" class="Bool"("Visible"=w473) -> ()  [unwired: 2 in, 2 out]
            n212 = property on="WG4 DL" class="Bool"("Visible"=FALSE) -> ()  [unwired: 2 in, 2 out]
          }
          frame #8 {
            w480 = 7205
            # "WG5 Vout\nAntenna"
            n213 = call "OpenChannel.vi"("error in (no error)"=w482, "Channel ID"=w480) -> ("error out"=w481:errorcluster)  [unwired: 1 in]
            n214 = Wait (ms)(milliseconds to wait=u32 500) -> ()  [unwired: 1 out]
          }
          frame #9 {
            n215 = call "Verify_Single.vi"("error in"=w489, "Switch ID"=w488, "Switch Functin"=enum16{"Open Switch", "Closed Switch"}."Open Switch") -> ("Error out"=w484:errorcluster, "Verfied"=w486:bool)  [unwired: 7 in]
            n216 = property on="WG5 ANT" class="Bool"("Visible"=w486) -> ()  [unwired: 2 in, 2 out]
            n217 = property on="WG5 DL" class="Bool"("Visible"=FALSE) -> ()  [unwired: 2 in, 2 out]
          }
        }
        n218 = flat-sequence {
          tunnel: w394 -> [w431]
          tunnel: [w431] -> w393
          tunnel: w392 -> [w430]
          tunnel: [w425] -> w391
          frame #0 {
            # "Enable\nXmit"
            n219 = call "OpenChannel.vi"("error in (no error)"=w430, "Channel ID"=7221) -> ("error out"=w426:errorcluster)  [unwired: 1 in]
            n220 = call "Verify_Single.vi"("error in"=w426, "Switch ID"=7221, "Switch Functin"=enum16{"Open Switch", "Closed Switch"}."Open Switch") -> ("Error out"=w425:errorcluster, "Verfied"=w424:bool)  [unwired: 7 in]
            n221 = Not(x=w424) -> (.not. x?=w423:bool)
            n222 = local write "XmStat"(w423) -> ()
          }
        }
        n223 = Release Queue(queue=w393, error in (no error)=w391) -> ()  [unwired: 1 in, 3 out]
      }
    }
  }
  n224 = while {
    tunnel: w5 -> [w494]
    tunnel: w3 -> [w493]
    stop <- w491 stop-if-true
    n225 = event shown="[5] \"Stop\": Value Change" {
      selector: _ -> [_ _ _ _ _ _ _]
      dyn-events: _ -> [_ _ _ _ _ _ _]
      timeout: 1000 -> [_ _ _ _ _ _ _]
      tunnel: w494 -> [w499 w504 w509 w514 w518 w522 w532]
      tunnel: w493 -> [w498 w503 w508 w513 w517 w524 w528]
      tunnel: [w497 w502 w507 w512 w516 w527 w530] -> _
      tunnel: [FALSE FALSE FALSE FALSE FALSE ("status") FALSE w531] -> w491
      event #0 {
        w495 = "Calibrate" ("element")
        n226 = event-data() -> ()  [unwired: 1 in, 1 out]
        n227 = Enqueue Element(queue=w499, element=w495, error in (no error)=w498) -> (error out=w497:errorcluster)  [unwired: 1 in, 2 out]
        n228 = local write "P-State"(w495) -> ()
      }
      event #1 {
        w500 = "Switches" ("element")
        n229 = event-data() -> ()  [unwired: 1 in, 1 out]
        n230 = Enqueue Element(queue=w504, element=w500, error in (no error)=w503) -> (error out=w502:errorcluster)  [unwired: 1 in, 2 out]
        n231 = local write "P-State"(w500) -> ()
      }
      event #2 {
        w505 = "121 dB" ("element")
        n232 = event-data() -> ()  [unwired: 1 in, 1 out]
        n233 = Enqueue Element(queue=w509, element=w505, error in (no error)=w508) -> (error out=w507:errorcluster)  [unwired: 1 in, 2 out]
        n234 = local write "P-State"(w505) -> ()
      }
      event #3 {
        w510 = "70 dB" ("element")
        n235 = event-data() -> ()  [unwired: 1 in, 1 out]
        n236 = Enqueue Element(queue=w514, element=w510, error in (no error)=w513) -> (error out=w512:errorcluster)  [unwired: 1 in, 2 out]
        n237 = local write "P-State"(w510) -> ()
      }
      event #4 {
        w519 = "Configuration 1" ("element")
        n238 = event-data() -> ()  [unwired: 1 in, 3 out]
        n239 = Enqueue Element(queue=w518, element=w519, error in (no error)=w517) -> (error out=w516:errorcluster)  [unwired: 1 in, 2 out]
        n240 = local write "P-State"(w519) -> ()
      }
      event #5 {
        w525 = "Stop" ("element")
        n241 = event-data() -> ()  [unwired: 1 in, 1 out]
        n242 = Enqueue Element(queue=w522, element="Initialize", error in (no error)=w524) -> (queue out=w521:refnum<queue>, error out=w523:errorcluster)  [unwired: 1 in, 1 out]
        n243 = Enqueue Element(queue=w521, element=w525, error in (no error)=w523) -> (error out=w527:errorcluster)  [unwired: 1 in, 2 out]
        n244 = local write "P-State"(w525) -> ()
      }
      event #6 {
        n245 = event-data() -> ()  [unwired: 1 in, 1 out]
        n246 = Get Queue Status(queue=w532, error in (no error)=w528) -> (error out=w530:errorcluster)  [unwired: 1 in, 7 out]
        n247 = Unbundle By Name(w530) -> ("status"=w531:bool)
        "P-State" <- "Timeout" ("element")
      }
    }
  }
  "Instructions" <- "Noise Source Dummy Load Calibration\n\n1 - Disable or turn off transmitter\n2 - Stow Antenna (point vertically)\n3 - Turn off all florescnt lights\n3 - Start the labview program by clicking the Run arrow\n     (left most button under  drop down menues)\n     start cycle time about 35 seconds\n4 - Wait for the red 'BUSY' light to change to green 'READY'\n     All the control buttons on the control panel are active.\n5 - Select the noise source, its state (ON/OFF) and the wave\n     guide termination.\n6 - Calibrate with the red  'Calibrate' button\n      calibration cycle time is less than 1 minute\n7 - Exit the program with the red 'EXIT' button\n      exit cycle time about 20 seconds\n\nHints:\nWait for the green 'READY' light before clicking buttons\nAll the status leds on the 'Status' tab should be green during a calibration.\nThe antenna noise source does not work with the wave guide\ntermination in the 'Dummy Load' position." ("String")
  "XmStat" <- w1
